vi "AnalyzeVIs.vi"(8 "error in (no error)":errorcluster) -> (0 "error out":errorcluster)   [LabVIEW 2020, in "CICD.lvlib"]
doc: "Run VI Analyzer."
uses:
  CICD.lvlib
  Private/Scope--enum.ctl
  <vilib>/Wiresmith Technology/G CLI/Argument Parser/Option Class/Option Configuration.ctl
  <vilib>/Wiresmith Technology/G CLI/Argument Parser/Option Class/Argument Type.ctl
  <vilib>/Wiresmith Technology/G CLI/CLI Class/CLI.lvclass
  <vilib>/Wiresmith Technology/G CLI/Argument Parser/Option Set Class/Option Set.lvclass
  <vilib>/Wiresmith Technology/G CLI/Argument Parser/Option Class/Option.lvclass
panel:
  out "-Scope":T1
  out "Output -ReportPath":path
  out "VIAnalyzer -ConfigPath":path
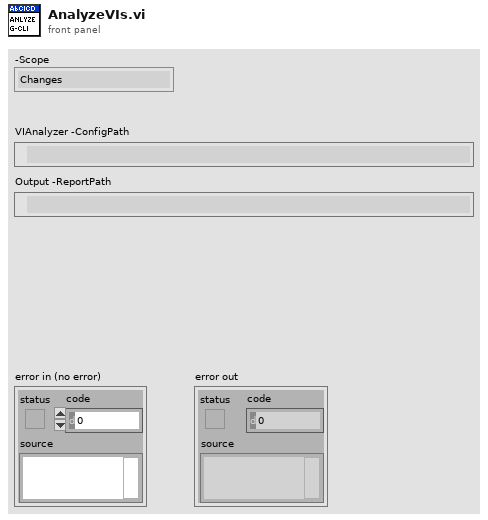
[diagram p1: front panel]
types:
  T1 = typedef "CICD.lvlib/Scope--enum.ctl" = enum16{"Changes", "All", "Folder"}
  T2 = typedef "Option Parser.lvlib/Option.lvclass/Option Configuration.ctl" = cluster{"Option Type":T3, "Option Labels":string[], "Key":string, "Description":string, "Required":bool, "Default Value":string}
  T3 = typedef "Option Parser.lvlib/Option.lvclass/Argument Type.ctl" = enum16{"flag", "value"}
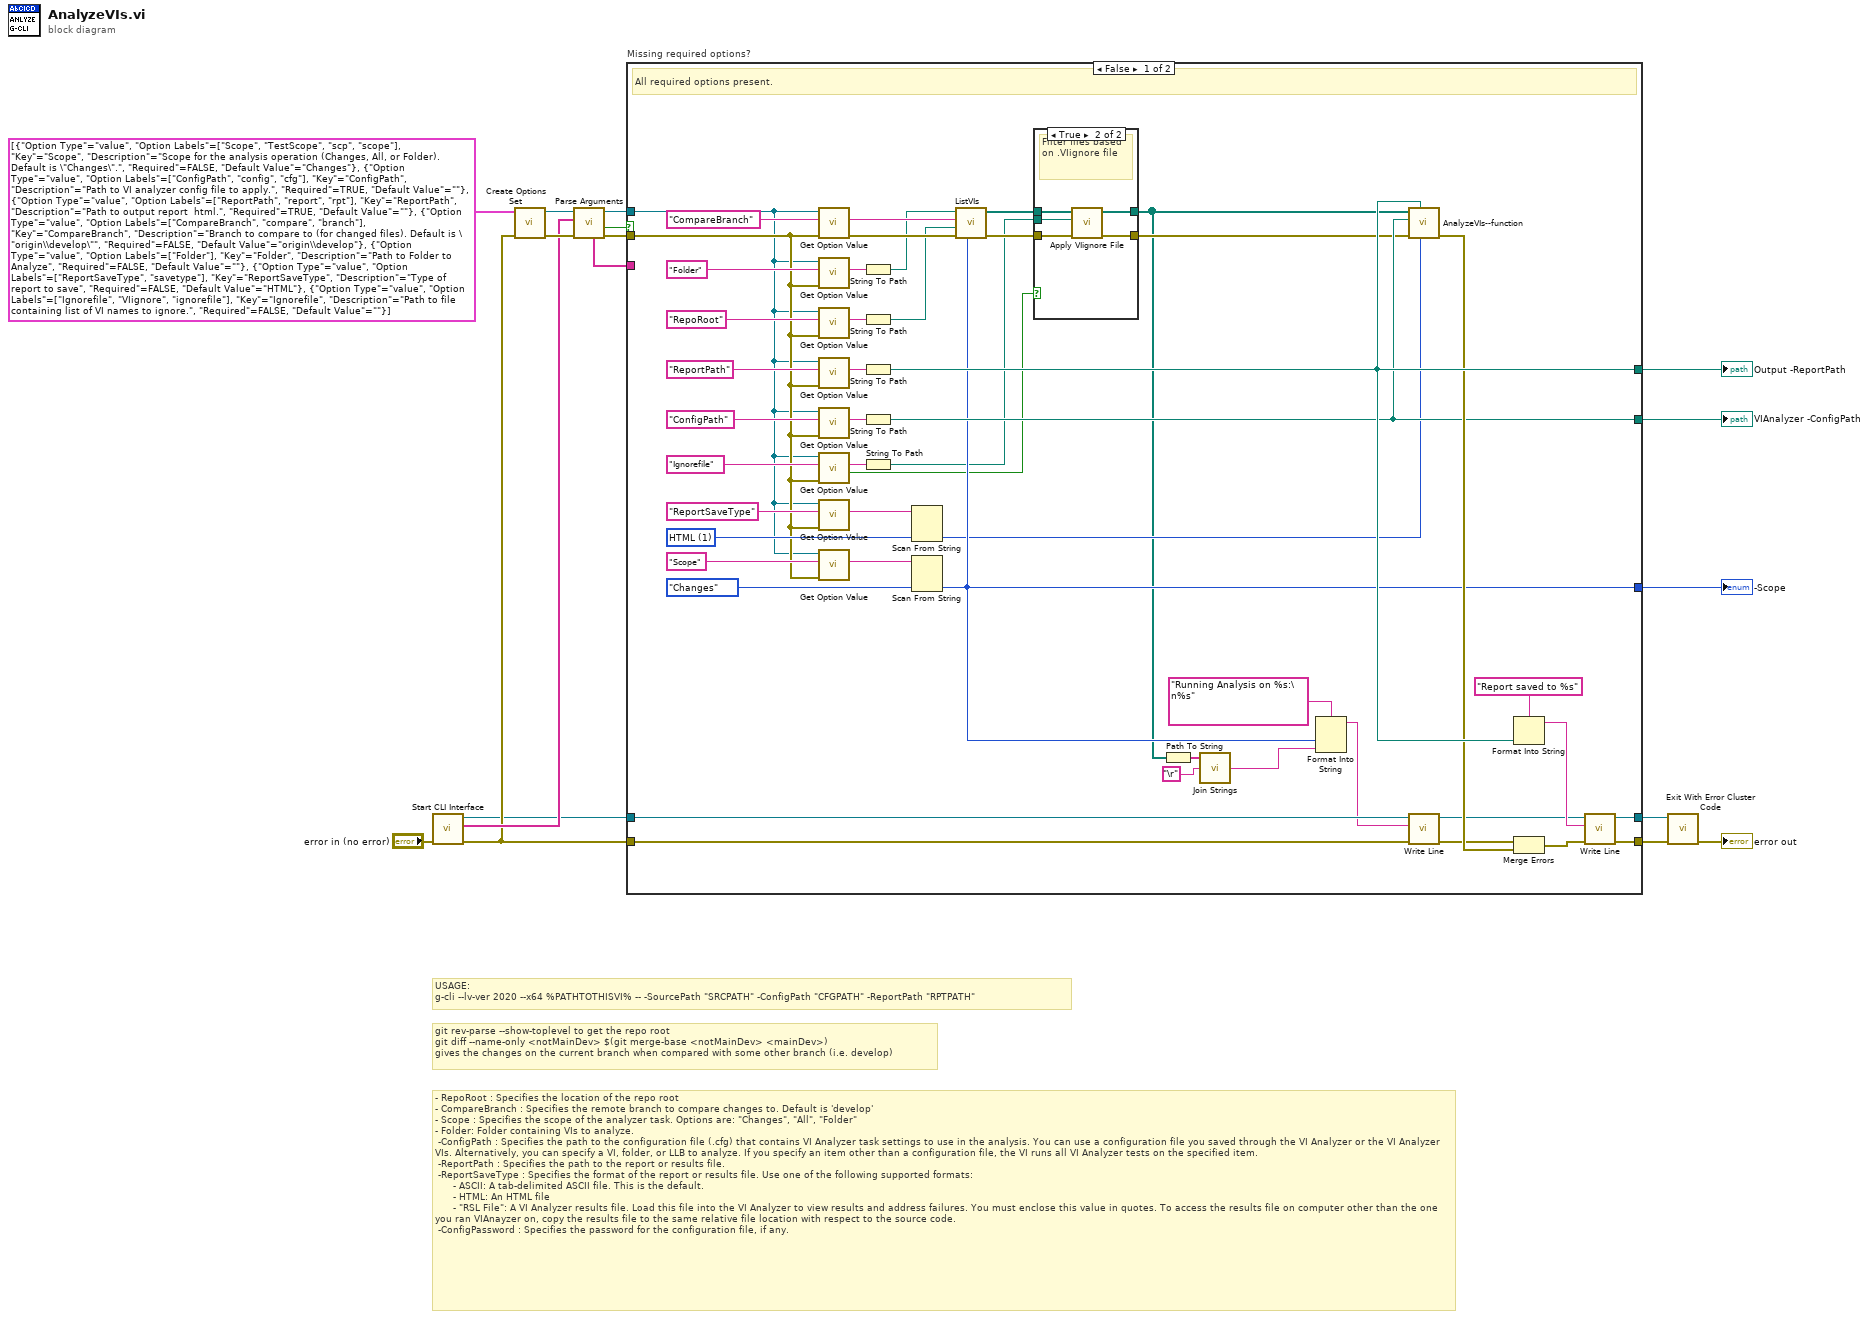
[diagram p0: block diagram]
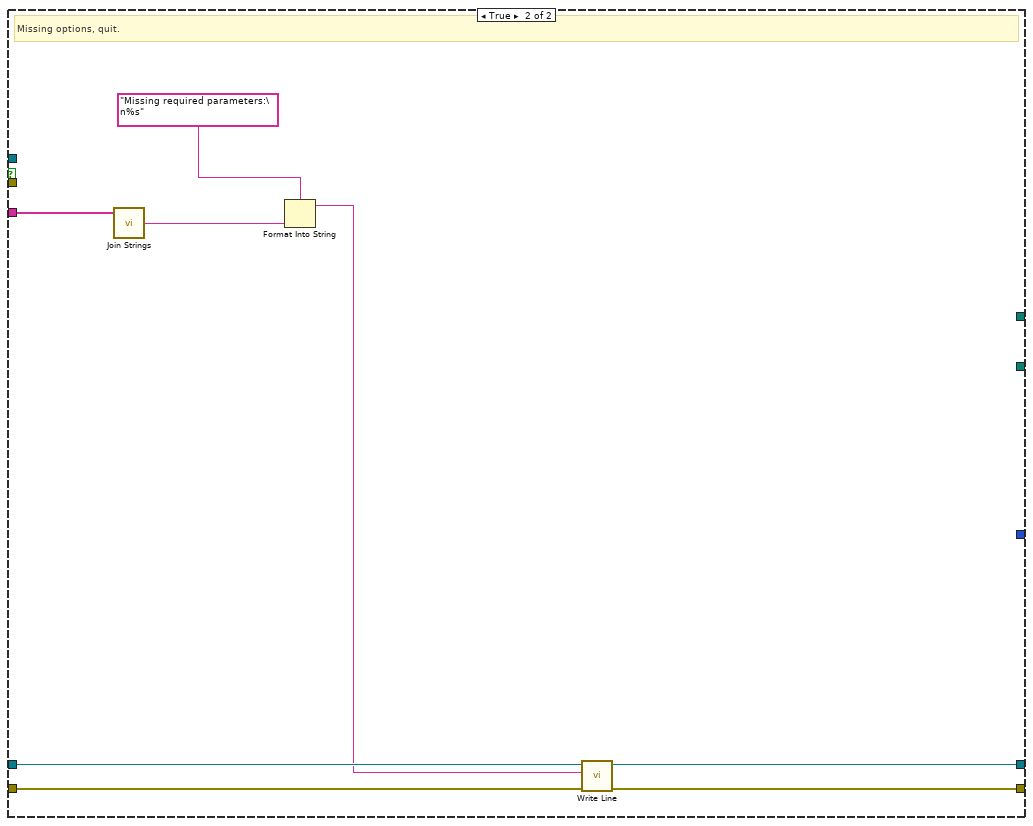
[diagram p3: hidden frame]
diagram:
  # "- RepoRoot : Specifies the location of the repo root\n- CompareBranch : Specifies the remote branch to compare changes to. Default is 'develop'\n- Scope : Specifies the scope of the analyzer task. Options are: \"Changes\", \"All\", \"Folder\"\n- Folder: Folder containing VIs to analyze.\n -ConfigPath : Specifies the path to the configuration file (.cfg) that contains VI Analyzer task settings to use in the analysis. You can use a configuration file you saved through the VI Analyzer or the VI Analyzer VIs. Alternatively, you can specify a VI, folder, or LLB to analyze. If you specify an item other than a configuration file, the VI runs all VI Analyzer tests on the specified item.\n -ReportPath : Specifies the path to the report or results file. \n -ReportSaveType : Specifies the format of the report or results file. Use one of the following supported formats:\n      - ASCII: A tab-delimited ASCII file. This is the default.\n      - HTML: An HTML file\n      - \"RSL File\": A VI Analyzer results file. Load this file into the VI Analyzer to view results and address failures. You must enclose this value in quotes. To access the results file on computer other than the one you ran VIAnayzer on, copy the results file to the same relative file location with respect to the source code.\n -ConfigPassword : Specifies the password for the configuration file, if any."
  # "git rev-parse --show-toplevel to get the repo root\ngit diff --name-only <notMainDev> $(git merge-base <notMainDev> <mainDev>)\ngives the changes on the current branch when compared with some other branch (i.e. develop)"
  # "USAGE:\ng-cli --lv-ver 2020 --x64 %PATHTOTHISVI% -- -SourcePath \"SRCPATH\" -ConfigPath \"CFGPATH\" -ReportPath \"RPTPATH\""
  n1 = call <vilib>:"Start CLI Interface.vi"("error in (no error)"="error in (no error)") -> ("error out"=w7:errorcluster, "Custom Parameters"=w12:string[], "CLI out"=w6:refnum<class "CLI.lvclass">)  [unwired: 7 in, 1 out]
  n2 = call <vilib>:"Create Options Set.vi"("error in (no error)"=w7, "Options"=T2[] [{"Option Type"=enum."value", "Option Labels"=["Scope", "TestScope", "scp", "scope"], "Key"="Scope", "Description"="Scope for the analysis operation (Changes, All, or Folder). Default is \"Changes\".", "Required"=FALSE, "Default Value"="Changes"}, {"Option Type"=enum."value", "Option Labels"=["ConfigPath", "config", "cfg"], "Key"="ConfigPath", "Description"="Path to VI analyzer config file to apply.", "Required"=TRUE, "Default Value"=""}, {"Option Type"=enum."value", "Option Labels"=["ReportPath", "report", "rpt"], "Key"="ReportPath", "Description"="Path to output report  html.", "Required"=TRUE, "Default Value"=""}, {"Option Type"=enum."value", "Option Labels"=["CompareBranch", "compare", "branch"], "Key"="CompareBranch", "Description"="Branch to compare to (for changed files). Default is \"origin\\develop\"", "Required"=FALSE, "Default Value"="origin\\develop"}, {"Option Type"=enum."value", "Option Labels"=["Folder"], "Key"="Folder", "Description"="Path to Folder to Analyze", "Required"=FALSE, "Default Value"=""}, {"Option Type"=enum."value", "Option Labels"=["ReportSaveType", "savetype"], "Key"="ReportSaveType", "Description"="Type of report to save", "Required"=FALSE, "Default Value"="HTML"}, {"Option Type"=enum."value", "Option Labels"=["Ignorefile", "VIignore", "ignorefile"], "Key"="Ignorefile", "Description"="Path to file containing list of VI names to ignore.", "Required"=FALSE, "Default Value"=""}]) -> ("error out"=w13:errorcluster, "Option Set out"=w14:refnum<class "Option Set.lvclass">)  [unwired: 8 in]
  n3 = call <vilib>:"Parse Arguments.vi"("error in (no error)"=w13, "Arguments"=w12, "Option Set in"=w14) -> ("error out"=w10:errorcluster, "Missing Options"=w8:bool, "Option Set out"=w11:refnum<class "Option Set.lvclass">, "Missing Option Keys"=w3:string[])  [unwired: 5 in]
  n4 = case "Missing required options?" shown="False" w8 {
    tunnel: [w57 w79] -> w16
    tunnel: w11 -> [w24 _]
    tunnel: w10 -> [w25 _]
    tunnel: w7 -> [w59 w80]
    tunnel: w6 -> [w56 w78]
    tunnel: [w53 _] -> w5
    tunnel: [w37 _] -> w4
    tunnel: w3 -> [_ w76]
    tunnel: [w52 w73] -> w2
    tunnel: [w31 _] -> w1
    frame False {
      w29 = u16 1 items=["ASCII", "HTML", "RSL File"] ("Report Save Type (ASCII)")
      # "All required options present."
      n5 = call <vilib>:"Get Option Value.vi"("error in (no error)"=w25, "Option Key"="CompareBranch", "Option Set in"=w24) -> ("error out"=w48:errorcluster, "Value"=w42:string)  [unwired: 5 in, 2 out]
      n6 = call <vilib>:"Get Option Value.vi"("error in (no error)"=w25, "Option Key"="Folder", "Option Set in"=w24) -> ("Value"=w63:string)  [unwired: 5 in, 3 out]
      n7 = call <vilib>:"Get Option Value.vi"("error in (no error)"=w25, "Option Key"="RepoRoot", "Option Set in"=w24) -> ("Value"=w34:string)  [unwired: 5 in, 3 out]
      n8 = call <vilib>:"Get Option Value.vi"("error in (no error)"=w25, "Option Key"="ReportPath", "Option Set in"=w24) -> ("Value"=w62:string)  [unwired: 5 in, 3 out]
      n9 = call <vilib>:"Get Option Value.vi"("error in (no error)"=w25, "Option Key"="ConfigPath", "Option Set in"=w24) -> ("Value"=w38:string)  [unwired: 5 in, 3 out]
      n10 = call <vilib>:"Get Option Value.vi"("error in (no error)"=w25, "Option Key"="Ignorefile", "Option Set in"=w24) -> ("Set"=w19:bool, "Value"=w23:string)  [unwired: 5 in, 2 out]
      n11 = call <vilib>:"Get Option Value.vi"("error in (no error)"=w25, "Option Key"="ReportSaveType", "Option Set in"=w24) -> ("Value"=w28:string)  [unwired: 5 in, 3 out]
      n12 = call <vilib>:"Get Option Value.vi"("error in (no error)"=w25, "Option Key"="Scope", "Option Set in"=w24) -> ("Value"=w36:string)  [unwired: 5 in, 3 out]
      n13 = String To Path(string=w63) -> (path=w39:path)
      n14 = String To Path(string=w34) -> (path=w33:path)
      n15 = String To Path(string=w62) -> (path=w53:path)
      n16 = String To Path(string=w38) -> (path=w37:path)
      n17 = String To Path(string=w23) -> (path=w18:path)
      n18 = Scan From String(input string=w28, default 1=w29) -> (output 1=w27:u16)  [unwired: 3 in, 3 out]
      n19 = Scan From String(input string=w36, default 1=Scope--enum."Changes" ("-TestScope")) -> (output 1=w31:T1)  [unwired: 3 in, 3 out]
      n20 = call "ListVIs.vi"("Scope"=w31, "error in"=w48, "RepoRoot"=w33, "Remote Branch to Compare"=w42, "Folder Path"=w39) -> ("error out"=w54:errorcluster, "VIs"=w21:path[])  [unwired: 5 in]
      n21 = case shown="True" w19 {
        tunnel: w54 -> [w67 w72]
        tunnel: [w67 w71] -> w22
        tunnel: w21 -> [w66 w70]
        tunnel: [w66 w69] -> w20
        tunnel: w18 -> [_ w68]
        frame False {
        }
        frame True {
          # "Filter files based on .VIignore file"
          n22 = call "Apply VIignore File.vi"("error in"=w72, ".VIignore file"=w68, "VI paths in"=w70) -> ("error out"=w71:errorcluster, "VI paths filtered"=w69:path[])  [unwired: 6 in, 1 out]
        }
      }
      n23 = Path To String(path=w20) -> (string=w45:string[])
      n24 = call <vilib>:"Join Strings.vi"("Separator (,)"="\r", "Strings In"=w45) -> ("String"=w41:string)  [unwired: 1 in]
      n25 = Format Into String(format string="Running Analysis on %s:\n%s", w31, w41) -> (resulting string=w32:string)  [unwired: 2 in, 1 out]
      n26 = call "AnalyzeVIs--function.vi"("Report Save Type (ASCII)"=w27, "ReportPath"=w53, "error in"=w22, "VIANConfig"=w37, "VIs to Analyze"=w20) -> ("error out"=w50:errorcluster)  [unwired: 5 in, 1 out]
      n27 = call <vilib>:"Write Line.vi"("error in (no error)"=w59, "Text to Write"=w32, "CLI in"=w56) -> ("error out"=w47:errorcluster, "CLI out"=w46:refnum<class "CLI.lvclass">)  [unwired: 7 in]
      n28 = Format Into String(format string="Report saved to %s", w53) -> (resulting string=w49:string)  [unwired: 2 in, 1 out]
      n29 = Merge Errors(w47, w50) -> (w51:errorcluster)
      n30 = call <vilib>:"Write Line.vi"("error in (no error)"=w51, "Text to Write"=w49, "CLI in"=w46) -> ("error out"=w57:errorcluster, "CLI out"=w52:refnum<class "CLI.lvclass">)  [unwired: 7 in]
    }
    frame True {
      # "Missing options, quit."
      n31 = call <vilib>:"Join Strings.vi"("Strings In"=w76) -> ("String"=w77:string)  [unwired: 2 in]
      n32 = Format Into String(format string="Missing required parameters:\n%s" ("Text to Write"), w77) -> (resulting string=w74:string)  [unwired: 2 in, 1 out]
      n33 = call <vilib>:"Write Line.vi"("error in (no error)"=w80, "Text to Write"=w74, "CLI in"=w78) -> ("error out"=w79:errorcluster, "CLI out"=w73:refnum<class "CLI.lvclass">)  [unwired: 7 in]
    }
  }
  "VIAnalyzer -ConfigPath" <- w4
  "Output -ReportPath" <- w5
  "-Scope" <- w1
  n34 = call <vilib>:"Exit With Error Cluster Code.vi"("error in (no error)"=w16, "CLI in"=w2) -> ("error out"=→"error out":errorcluster)  [unwired: 9 in]
